vi "taller_3.vi"() -> ()   [LabVIEW 2023]
panel:
  in  "Válvula":u16(ring) items=["Lineal", "Isoporcentual", "Apertura Rápida"]
  in  "dt":dbl min=0.0 step=0.5
  in  "Stop Button":bool
  out "Nivel":dbl
  in  "h_t-1":dbl min=0.0 step=0.1
  in  "Área":dbl min=0.0 step=1.0
  in  "Alpha":dbl=10.0 min=10.0 max=100.0 step=10.0
  in  "a2":dbl min=0.0 max=1.0 step=0.1
  in  "a1":dbl min=0.0 max=1.0 step=0.1
  in  "k2":dbl min=0.0 step=0.01
  in  "k1":dbl min=0.0 step=0.01
  out "h_t":dbl(slide) scale=0.0..20.0
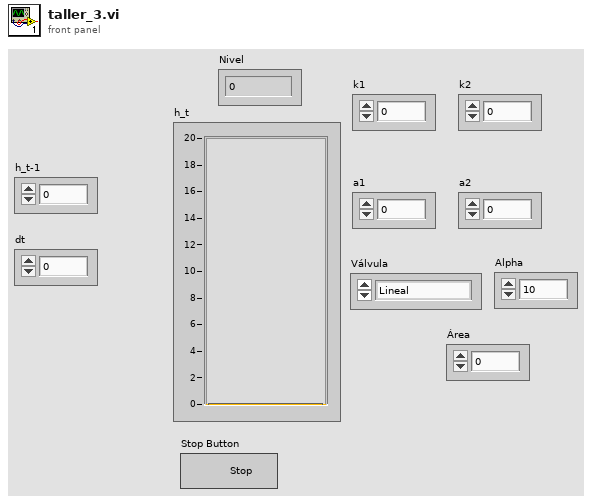
[diagram p1: front panel]
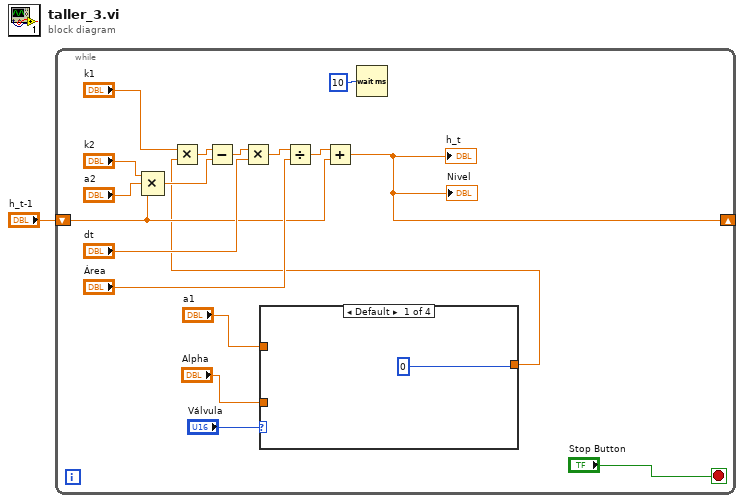
[diagram p0: block diagram]
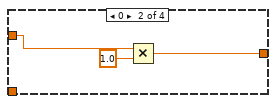
[diagram p2: hidden frame]
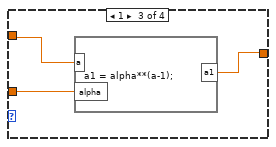
[diagram p3: hidden frame]
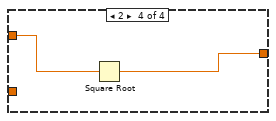
[diagram p4: hidden frame]
diagram:
  n1 = while {
    shift-right: [w6] -> _
    shift-left: "h_t-1" -> [w7]
    stop <- "Stop Button" stop-if-true
    n2 = Compound Arithmetic op=MULTIPLY("k2", "a2", w7) -> (w14:dbl)
    n3 = case shown="Default" "Válvula" {
      tunnel: "a1" -> [_ w23 w25 w28]
      tunnel: [0 w22 w24 w27] -> w3
      tunnel: "Alpha" -> [_ _ w26 _]
      frame Default {
      }
      frame 0 {
        n4 = Multiply(x=w23, y=1.0) -> (x*y=w22:dbl)
      }
      frame 1 {
        n5 = formula code="a1 = alpha**(a-1);"("a"=w25, "alpha"=w26) -> ("a1"=w24:dbl)
      }
      frame 2 {
        n6 = Square Root(x=w28) -> (sqrt(x)=w27:dbl)
      }
    }
    n7 = Multiply(x="k1", y=w3) -> (x*y=w15:dbl)
    n8 = Subtract(x=w15, y=w14) -> (x-y=w12:dbl)
    n9 = Multiply(x=w12, y="dt") -> (x*y=w11:dbl)
    n10 = Divide(x=w11, y="Área") -> (x/y=w9:dbl)
    n11 = Add(x=w9, y=w7) -> (x+y=w6:dbl)
    "h_t" <- w6
    "Nivel" <- w6
    n12 = Wait (ms)(milliseconds to wait=u32 10) -> ()  [unwired: 1 out]
  }
